vi "write_FXP_18-5_data_to_fpga.vi"(8 "error in":errorcluster, 10 "all rows":fxp<+/-,18,5>[](array[numeric]), 11 "FPGA Interface":T1) -> (0 "error out":errorcluster, 3 "elements left":i32=1)   [LabVIEW 2017, in "fpga_interface.lvlib"]
uses:
  fpga_interface.lvlib
  fpga_interface_types/HOST_to_FPGA_FXP_18-5_FIFO_interface.ctl
  <vilib>/Utility/error.llb/Error Cluster From Error Code.vi
  <vilib>/rvi/errors/niLvFpgaAdjustHostInterfaceError.vi
  <vilib>/rvi/interface/nirviMethod/nirviMethod.xnode
  <vilib>/FPGAPlugInAG/Dynamic/niLvFpga_WriteFifo_Dynamic.vi
  <vilib>/rvi/errors/niLvFpgaMergeErrorWithErrorCode.vi
panel:
  out "Numeric":i32
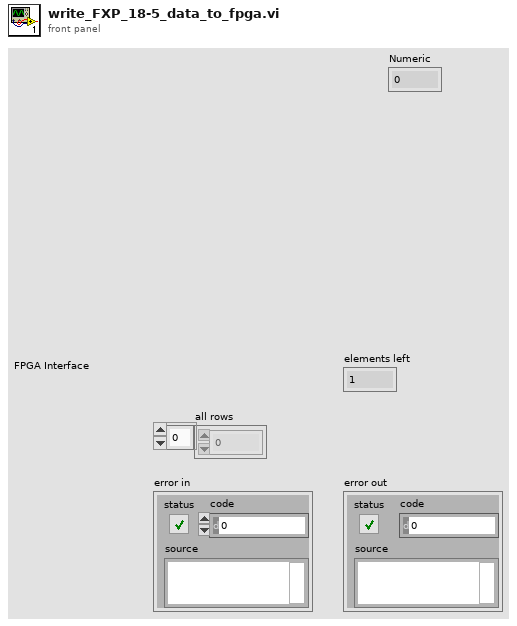
[diagram p1: front panel]
types:
  T1 = typedef "fpga_interface.lvlib/HOST_to_FPGA_FXP_18-5_FIFO_interface.ctl" = refnum<k20>
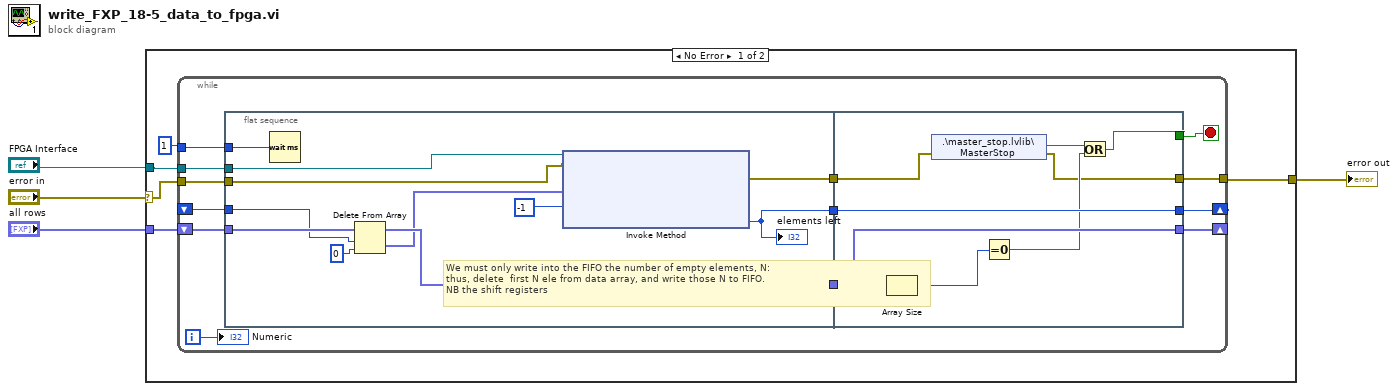
[diagram p0: block diagram]
diagram:
  n1 = case shown="No Error" "error in" {
    selector: "error in" -> [w5 w42]
    tunnel: [w9 w42] -> w4
    tunnel: "all rows" -> [w8 _]
    tunnel: "FPGA Interface" -> [w6 _]
    frame No Error {
      n2 = while {
        tunnel: [w20] -> w9
        tunnel: 1 -> [w22]
        shift-right: [w15] -> _
        shift-left: _ -> [w19]
        shift-right: [w13] -> _
        shift-left: w8 -> [w21]
        tunnel: w6 -> [w12]
        tunnel: w5 -> [w11]
        i -> [w10]
        stop <- w16 stop-if-true
        n3 = flat-sequence {
          tunnel: w22 -> [w33]
          tunnel: w21 -> [w30]
          tunnel: w19 -> [w29]
          tunnel: [w27] -> w18
          tunnel: [w24] -> w17
          tunnel: [w31] -> w14
          tunnel: w12 -> [w28]
          tunnel: w11 -> [w26]
          tunnel: [w41] -> w15
          tunnel: [w34] -> w20
          tunnel: w18 -> [w35]
          tunnel: w17 -> [w41]
          tunnel: [w37] -> w16
          tunnel: w14 -> [w39]
          tunnel: [w39] -> w13
          frame #0 {
            # "We must only write into the FIFO the number of empty elements, N:\nthus, delete  first N ele from data array, and write those N to FIFO.\nNB the shift registers"
            n4 = Wait (ms)(milliseconds to wait=w33) -> ()  [unwired: 1 out]
            n5 = Delete From Array(array=w30, length=w29, index=0) -> (deleted portion=w23:fxp<+/-,18,5>[], array with subset deleted=w31:fxp<+/-,18,5>[])
            n6 = xnode "Invoke Method"("FPGA VI Reference In"=w28, "error in"=w26, "Data"=w23, "Timeout (ms)"=-1) -> ("error out"=w27:errorcluster, "Empty Elements Remaining"=w24:u32)  [unwired: 1 out]
            "elements left" <- w24
          }
          frame #1 {
            n7 = Array Size(array=w39) -> (size(s)=w40:i32)
            n8 = shared-variable ".\\master_stop.lvlib\\MasterStop"(error in=w35) -> (w36:bool, error out=w34:errorcluster)
            n9 = Equal To 0?(x=w40) -> (x = 0?=w38:bool)
            n10 = Or(x=w36, y=w38) -> (x .or. y?=w37:bool)
          }
        }
        "Numeric" <- w10
      }
    }
    frame Error {
    }
  }
  "error out" <- w4
